vi "edittest parse permissions keys.vi"(4 "Test Station (F)":bool, 6 "Start with Changes? (f)":bool, 8 "error in (no error)":errorcluster, 9 "User Record":T2, 10 "Sequence Record":T1, 11 "Template Keys In (empty)":T3) -> (0 "error out":errorcluster, 3 "Template Keys Out":T3)   [LabVIEW 2011]
uses:
  ITK EXT/utils/keyedarr.llb/Keyed Array.ctl
  server/database/Users/User Record.ctl
  server/database/Sequences/Sequence Record.ctl
  ITK EXT/utils/strutil.llb/Case Matching.ctl
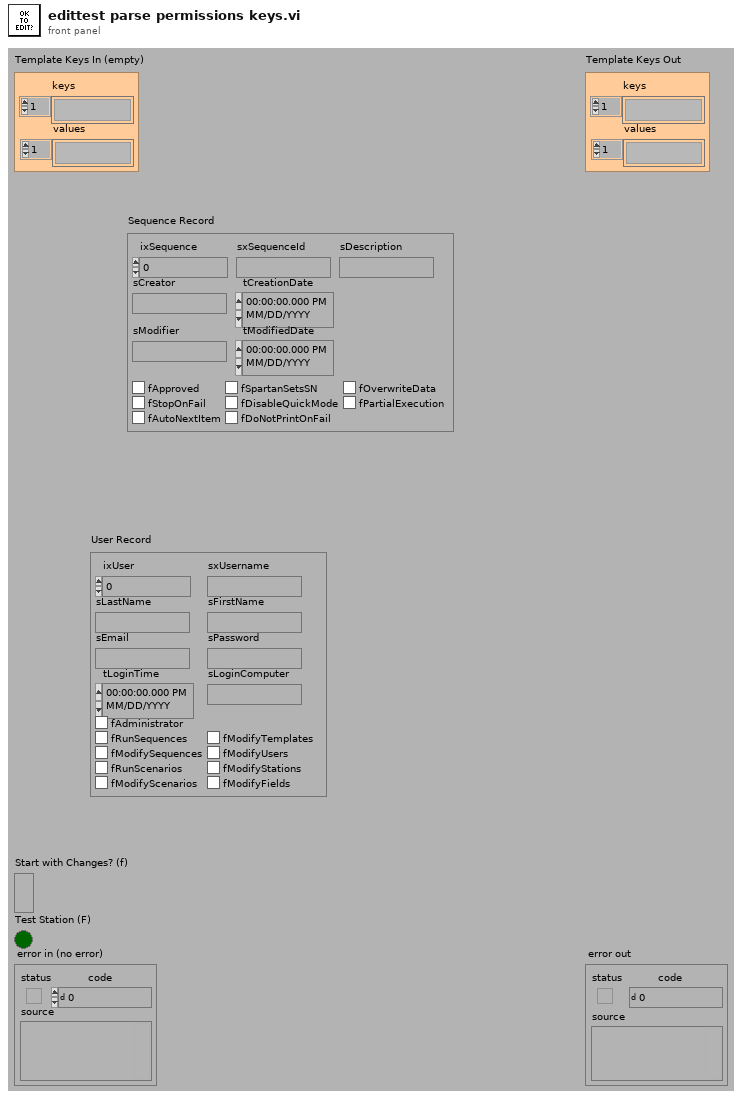
[diagram p1: front panel]
types:
  T1 = typedef "Sequence Record.ctl" = cluster{"ixSequence":i32, "sxSequenceId":string, "sDescription":string, "sCreator":string, "tCreationDate":timestamp, "sModifier":string, "tModifiedDate":timestamp, "fApproved":bool, "fSpartanSetsSN":bool, "fOverwriteData":bool, "fStopOnFail":bool, "fDisableQuickMode":bool, "fPartialExecution":bool, "fAutoNextItem":bool, "fDoNotPrintOnFail":bool}
  T2 = typedef "User Record.ctl" = cluster{"ixUser":i32, "sxUsername":string, "sLastName":string, "sFirstName":string, "sEmail":string, "sPassword":string, "tLoginTime":timestamp, "sLoginComputer":string, "fAdministrator":bool, "fRunSequences":bool, "fModifySequences":bool, "fRunScenarios":bool, "fModifyScenarios":bool, "fModifyTemplates":bool, "fModifyUsers":bool, "fModifyStations":bool, "fModifyFields":bool}
  T3 = typedef "Keyed Array.ctl" = cluster{"keys":string[], "values":string[]}
  T4 = typedef "Case Matching.ctl" = enum16{"a != A", "a == A", "system"}
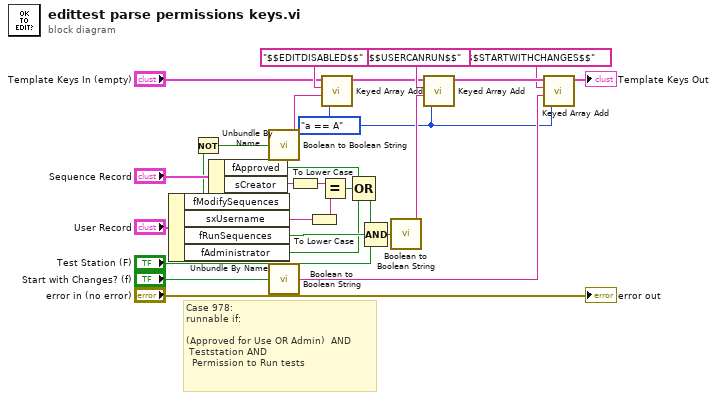
[diagram p0: block diagram]
diagram:
  w15 = Case_Matching."a == A" ("case matching (sensitive)")
  # "Case 978:\nrunnable if:\n\n(Approved for Use OR Admin)  AND\n Teststation AND\n  Permission to Run tests"
  n1 = Unbundle By Name("User Record") -> ("fModifySequences"=w1:bool, "sxUsername"=w4:string, "fRunSequences"=w12:bool, "fAdministrator"=w5:bool)
  n2 = Not(x=w1) -> (.not. x?=w24:bool)
  n3 = Unbundle By Name("Sequence Record") -> ("fApproved"=w2:bool, "sCreator"=w3:string)
  n4 = call "Boolean to Boolean String.vi"("Boolean"=w24) -> ("Boolean string"=w21:string)  [unwired: 1 in]
  n5 = call "Boolean to Boolean String.vi"("Boolean"="Start with Changes? (f)") -> ("Boolean string"=w20:string)  [unwired: 1 in]
  n6 = To Lower Case(string=w3) -> (all lower case string=w8:string)
  n7 = To Lower Case(string=w4) -> (all lower case string=w9:string)
  n8 = Equal?(x=w8, y=w9) -> (x = y?=w7:bool)
  n9 = call "Keyed Array Add.vi"("case matching (sensitive)"=w15, "value"=w21, "key"="$$EDITDISABLED$$", "array in"="Template Keys In (empty)") -> ("array out"=w26:T3)  [unwired: 3 out]
  n10 = Compound Arithmetic op=OR(w2, w7, w5) -> (w6:bool)
  n11 = Compound Arithmetic op=AND(w6, w12, "Test Station (F)") -> (w11:bool)
  n12 = call "Boolean to Boolean String.vi"("Boolean"=w11) -> ("Boolean string"=w23:string)  [unwired: 1 in]
  n13 = call "Keyed Array Add.vi"("case matching (sensitive)"=w15, "value"=w23, "key"="$$USERCANRUN$$", "array in"=w26) -> ("array out"=w19:T3)  [unwired: 3 out]
  n14 = call "Keyed Array Add.vi"("case matching (sensitive)"=w15, "value"=w20, "key"="$$STARTWITHCHANGES$$", "array in"=w19) -> ("array out"=→"Template Keys Out":T3)  [unwired: 3 out]
  "error out" <- "error in (no error)"
